vi "globals.vi"() -> ()   [LabVIEW 2017]
panel:
  out "exit":bool
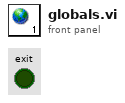
[diagram p1: front panel]
diagram:
